vi "Determine Input Matrix.vi"() -> ()   [LabVIEW 2014]
uses:
  <vilib>/Analysis/NI_AALPro.lvlib
  <vilib>/Analysis/polynomials.llb/nth Derivative of Polynomial (DBL).vi
  <vilib>/Analysis/polynomials.llb/nth Derivative of Rational Polynomial (DBL).vi
  Tag.lvclass
panel:
  in  "Werpkunt q":T1
  in  "Werpkunt p":T1
  out "yq":dbl
  out "xq":dbl
  out "yp":dbl
  out "xp":dbl
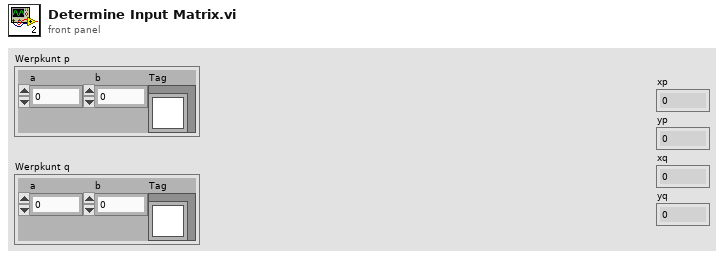
[diagram p1: front panel]
types:
  T1 = cluster{"a":dbl, "b":dbl, "Tag":refnum<class "Tag.lvclass">}
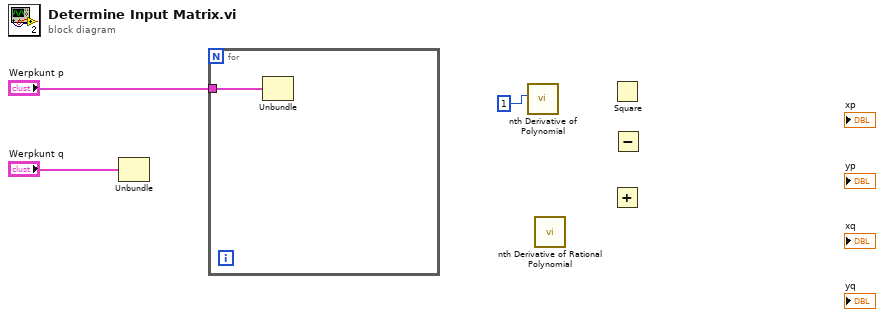
[diagram p0: block diagram]
diagram:
  n1 = Unbundle("Werpkunt q") -> ()  [unwired: 3 out]
  n2 = for {
    tunnel: "Werpkunt p" -> [w4]
    n3 = Unbundle(w4) -> ()  [unwired: 3 out]
  }
  n4 = call-poly <vilib>:"nth Derivative of Polynomial.vi"("order"=1) -> ()  [unwired: 9 in, 2 out]
  n5 = call-poly <vilib>:"nth Derivative of Rational Polynomial.vi"() -> ()  [unwired: 9 in, 3 out]
  n6 = Square() -> ()  [unwired: 1 in, 1 out]
  n7 = Add() -> ()  [unwired: 2 in, 1 out]
  n8 = Subtract() -> ()  [unwired: 2 in, 1 out]
